vi "Read Voltage From Channel.vi"(8 "Error In":errorcluster, 10 "Channel":u8, 11 "reference in":refnum<class "PXIe-5172Ref.lvclass">) -> (0 "Error Out":errorcluster, 2 "Voltage":dbl format="%#_g V", 3 "reference out":refnum<class "PXIe-5172Ref.lvclass">)   [LabVIEW 2023, in "PXIe-5172.lvlib" / "PXIe-5172Ref.lvclass"]
uses:
  PXIe-5172Ref.lvclass
  PXIe-5172.lvclass
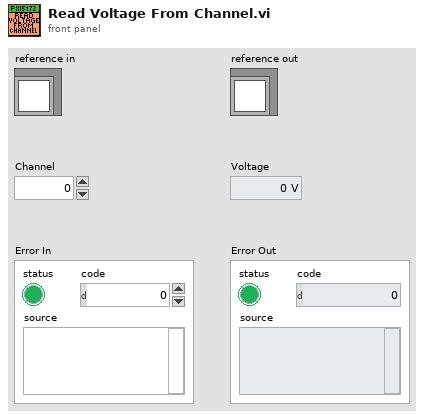
[diagram p1: front panel]
types:
  T1 = typedef "PXIe-5172.lvlib/PXIe-5172Ref.lvclass/ObjectAttributes.ctl" = cluster{"PXIe-5172.lvclass":refnum<class "PXIe-5172.lvclass">}
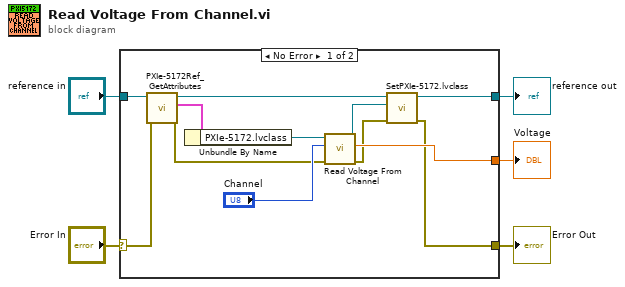
[diagram p0: block diagram]
diagram:
  n1 = case shown="No Error" "Error In" {
    selector: "Error In" -> [w17 w19]
    tunnel: [w7 w19] -> w4
    tunnel: [w6 w18] -> w2
    tunnel: "reference in" -> [w15 w18]
    tunnel: [w11 _] -> w1
    frame No Error {
      n2 = call "PXIe-5172Ref_GetAttributes.vi"("Error In"=w17, "reference in"=w15) -> ("Error Out"=w12:errorcluster, "Data"=w16:T1, "reference out"=w10:refnum<class "PXIe-5172Ref.lvclass">)  [unwired: 6 in, 1 out]
      n3 = Unbundle By Name(w16) -> ("PXIe-5172.lvclass"=w14:refnum<class "PXIe-5172.lvclass">)
      n4 = call-dynamic "Read Voltage From Channel.vi"("error in (no error)"=w12, "Channel"="Channel", "IRead Voltage Multichannel in"=w14) -> ("error out"=w9:errorcluster, "Voltage"=w11:dbl, "IRead Voltage Multichannel out"=w8:refnum<class "PXIe-5172.lvclass">)  [unwired: 6 in]
      n5 = call "SetPXIe-5172.lvclass.vi"("Error In"=w9, "PXIe-5172.lvclass"=w8, "reference in"=w10) -> ("Error Out"=w7:errorcluster, "reference out"=w6:refnum<class "PXIe-5172Ref.lvclass">)  [unwired: 7 in]
    }
    frame Error {
    }
  }
  "Error Out" <- w4
  "reference out" <- w2
  "Voltage" <- w1
